vi "checkBeginDirectEnemyPlay.vi"(8 "error in (no error)":errorcluster, 9 "last command_interpreted":T1, 10 "Game":refnum<class "Game.lvclass">, 11 "DirectEnemyPlay in":refnum<class "DirectEnemyPlay.lvclass">) -> (0 "error out":errorcluster, 2 "Boolean":bool, 3 "DirectEnemyPlay out":refnum<class "DirectEnemyPlay.lvclass">)   [LabVIEW 2023, in "DirectEnemyPlay.lvclass"]
uses:
  DirectEnemyPlay.lvclass
  Game_class/Game.lvclass
  Referee_class/command_interpreted.ctl
  Game_class/Game.lvclass/Game.ctl
  Referee_class/Referee.lvclass/Referee.ctl
  Game_class/Read Referee.vi
  Referee_class/Read command_interpreted.vi
  Referee_class/Referee.lvclass
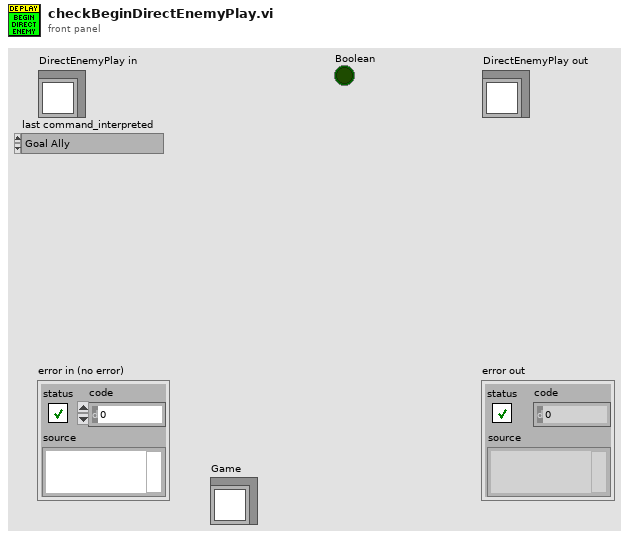
[diagram p1: front panel]
types:
  T1 = typedef "command_interpreted.ctl" = enum16{"Goal Ally", "Goal Enemy", "Ball Placement Enemy", "Ball Placement Ally", "Normal Half Time", "Extra Time  Break", "Extra Half Time", "None", "Post Game", "PKA Normal Start", "Prepare Kickoff Ally", "PKE Normal Start", "Prepare Kickoff Enemy", "Force Start", "Halt", "Timeout", "Prepare Penalty Ally", "Prepare Penalty Enemy", "PPA NormalStart", "PPE Normal Start", "Indirect Free Ally", "Direct Free Enemy", "Direct Free Ally", "Indirect Free Enemy", "Stop"}
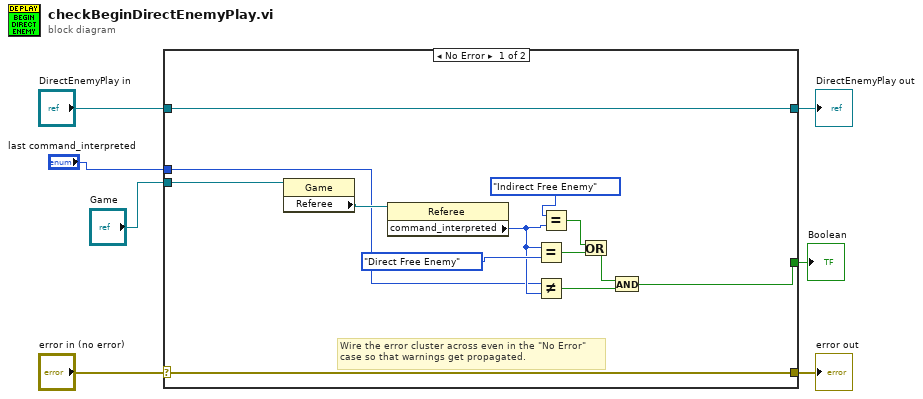
[diagram p0: block diagram]
diagram:
  n1 = case shown="No Error" "error in (no error)" {
    selector: "error in (no error)" -> [w19 w22]
    tunnel: [w19 w22] -> w6
    tunnel: [w20 w21] -> w4
    tunnel: "DirectEnemyPlay in" -> [w20 w21]
    tunnel: "Game" -> [w15 _]
    tunnel: [w14 _] -> w2
    tunnel: "last command_interpreted" -> [w8 _]
    frame No Error {
      # "Wire the error cluster across even in the \"No Error\"\ncase so that warnings get propagated."
      n2 = property class="Game"(reference=w15) -> ("Referee"=w18:refnum<class "Referee.lvclass">)  [unwired: 1 in, 2 out]
      n3 = property class="Referee"(reference=w18) -> ("command_interpreted"=w11:T1)  [unwired: 1 in, 2 out]
      n4 = Equal?(x=w11, y=command_interpreted."Direct Free Enemy" ("command_interpreted")) -> (x = y?=w12:bool)
      n5 = Not Equal?(x=w8, y=w11) -> (x != y?=w16:bool)
      n6 = Equal?(x=command_interpreted."Indirect Free Enemy" ("command_interpreted"), y=w11) -> (x = y?=w9:bool)
      n7 = Or(x=w9, y=w12) -> (x .or. y?=w13:bool)
      n8 = And(x=w13, y=w16) -> (x .and. y?=w14:bool)
    }
    frame Error {
    }
  }
  "error out" <- w6
  "DirectEnemyPlay out" <- w4
  "Boolean" <- w2
